vi "niScope Get Capabilities.vi"(8 "error in":errorcluster, 10 "fs [Hz]":dbl, 11 "niScope session in":T2={"channel cfg"=[], "sessions"=[], "multi cards"=FALSE, "channels"=0, "type"=enum."n/a", "memory [B/chn]"=0, "ext. clock [Hz]"=0.0, "samples count"=0, "use streaming"=FALSE, "proc setup"={"packet size [smpl]"=0, "current timeout [s]"=0.0, "blk2blk timeout [s]"=0.0, "event time"=timestamp(0 s since 1904-01-01), "temp sampl T [s]"=0.0, "data queue"=refnum, "stop notifier"=refnum, "proc ref"=refnum}, "sample width [B]"=0, "ranges [V]"=[], "trigger setup"={"coupling"=1, "level [V]"=0.0, "slope"=0, "mode"=enum."Immediate"}, "fs [Hz]"=0.0} {"trigger setup"."level [V]" format="%.2f"; "trigger setup"."coupling" items=["AC"=0, "DC"=1, "HF Reject"=3, "LF Reject"=4, "AC Plus HF Reject"=1001]; "channel cfg"."Range [Vpk]" min=0.0; "channel cfg"."Channel" min=0}) -> (0 "error out":errorcluster, 2 "capabilities":T1, 3 "niScope session out":T2={"channel cfg"=[], "sessions"=[], "multi cards"=FALSE, "channels"=0, "type"=enum."n/a", "memory [B/chn]"=0, "ext. clock [Hz]"=0.0, "samples count"=0, "use streaming"=FALSE, "proc setup"={"packet size [smpl]"=0, "current timeout [s]"=0.0, "blk2blk timeout [s]"=0.0, "event time"=timestamp(0 s since 1904-01-01), "temp sampl T [s]"=0.0, "data queue"=refnum, "stop notifier"=refnum, "proc ref"=refnum}, "sample width [B]"=0, "ranges [V]"=[], "trigger setup"={"coupling"=1, "level [V]"=0.0, "slope"=0, "mode"=enum."Immediate"}, "fs [Hz]"=0.0} {"trigger setup"."level [V]" format="%.2f"; "trigger setup"."coupling" items=["AC"=0, "DC"=1, "HF Reject"=3, "LF Reject"=4, "AC Plus HF Reject"=1001]; "channel cfg"."Range [Vpk]" min=0.0; "channel cfg"."Channel" min=0})   [LabVIEW 2013, in "niScope Virtual Digitizer.lvlib"]
doc: "This will return capabilities of selected HW. To make it work the session must contain valid setup of the channels and must also contain output of the 'Initialize Virtual Channels' VI, i.e. it may be calle either within opened session or even after the session was closed, because the data produced by 'Initialize Virtual Channels' stay in the session."
uses:
  niScope Virtual Digitizer.lvlib
  niScope Session.ctl
  niScope Virtual Channel Config.ctl
  niScope Virtual Channel Mode.ctl
  niScope Virtual Channel Input Z.ctl
  niScope Virtual Channel Coupling.ctl
  niScope Type.ctl
  niScope Digitizing Process Options.ctl
  niScope Data Packet.ctl
  niScope Trigger Setup.ctl
  <instrlib>/niScope/Controls/niScope trigger coupling.ctl
  <instrlib>/niScope/Controls/niScope trigger slope.ctl
  niScope Capabilities.ctl
  <vilib>/Utility/error.llb/Error Cluster From Error Code.vi
  <vilib>/ErrorRing/Error Ring.xnode
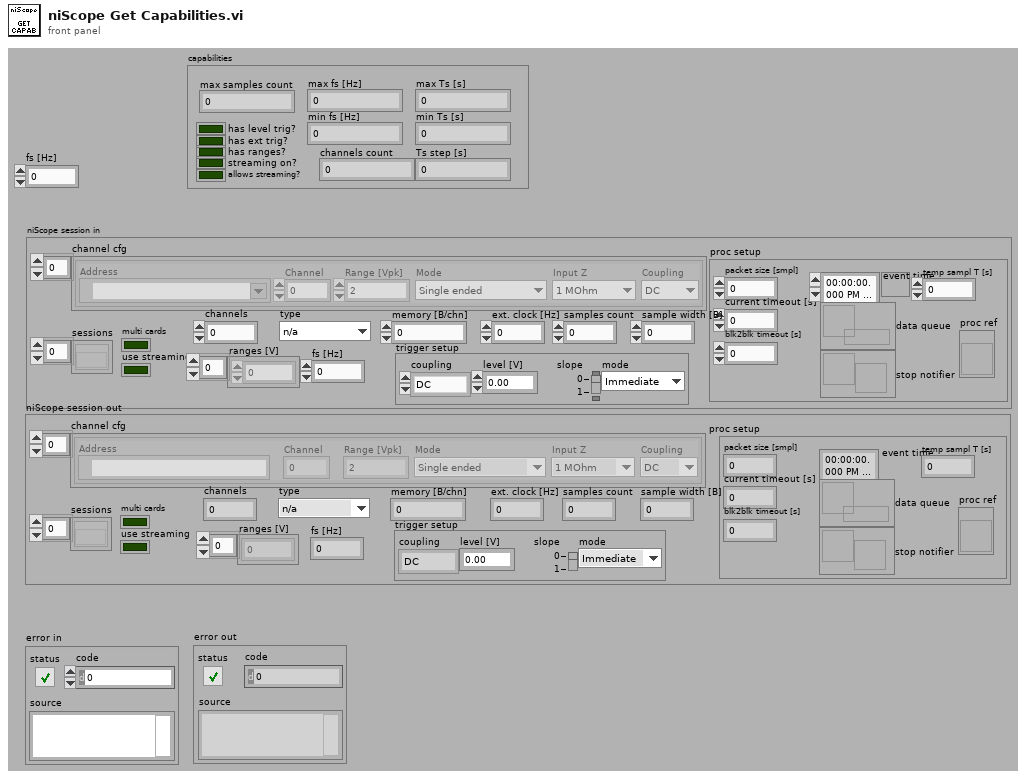
[diagram p1: front panel]
types:
  T1 = typedef "niScope Virtual Digitizer.lvlib/niScope Capabilities.ctl" = cluster{"max samples count":i64, "max fs [Hz]":ext, "min fs [Hz]":ext, "Ts step [s]":ext, "max Ts [s]":ext, "min Ts [s]":ext, "allows streaming?":bool, "streaming on?":bool, "has level trig?":bool, "has ext trig?":bool, "channels count":i32, "has ranges?":bool}
  T2 = typedef "niScope Virtual Digitizer.lvlib/niScope Session.ctl" = cluster{"channel cfg":T3[], "sessions":refnum<k20>[], "multi cards":bool, "channels":i32, "type":T7, "memory [B/chn]":i32, "ext. clock [Hz]":dbl, "samples count":i64, "use streaming":bool, "proc setup":T8, "sample width [B]":i32, "ranges [V]":dbl[], "trigger setup":T9, "fs [Hz]":dbl}
  T3 = typedef "niScope Virtual Digitizer.lvlib/niScope Virtual Channel Config.ctl" = cluster{"Address":refnum<k15>, "Channel":i32, "Mode":T4, "Input Z":T5, "Coupling":T6, "Range [Vpk]":dbl}
  T4 = typedef "niScope Virtual Digitizer.lvlib/niScope Virtual Channel Mode.ctl" = enum16{"Single ended", "Unbal. differential", "Differential"}
  T5 = typedef "niScope Virtual Digitizer.lvlib/niScope Virtual Channel Input Z.ctl" = enum16{"1 MOhm", "50 Ohm"}
  T6 = typedef "niScope Virtual Digitizer.lvlib/niScope Virtual Channel Coupling.ctl" = enum16{"AC", "DC", "GND"}
  T7 = typedef "niScope Virtual Digitizer.lvlib/niScope Type.ctl" = enum16{"n/a", "5922"}
  T8 = typedef "niScope Virtual Digitizer.lvlib/niScope Digitizing Process Options.ctl" = cluster{"packet size [smpl]":i64, "current timeout [s]":dbl, "blk2blk timeout [s]":dbl, "event time":timestamp, "temp sampl T [s]":dbl, "data queue":refnum<queue>, "stop notifier":refnum<notifier>, "proc ref":refnum<vi>}
  T9 = typedef "niScope Virtual Digitizer.lvlib/niScope Trigger Setup.ctl" = cluster{"coupling":T10, "level [V]":dbl, "slope":T11, "mode":enum16{"Immediate", "External", "Level"}}
  T10 = typedef "niScope trigger coupling.ctl" = u16
  T11 = typedef "niScope trigger slope.ctl" = i32
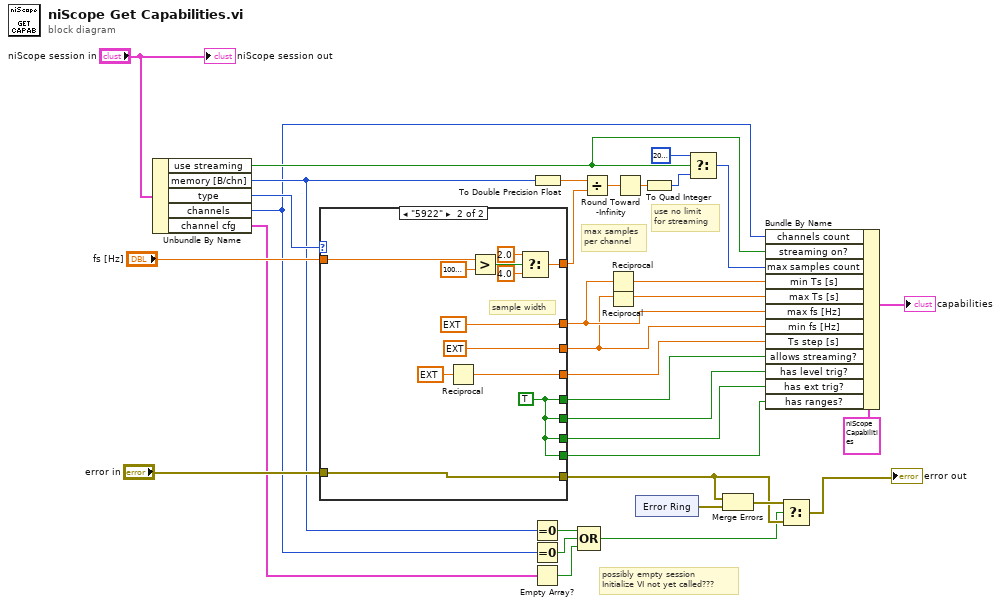
[diagram p0: block diagram]
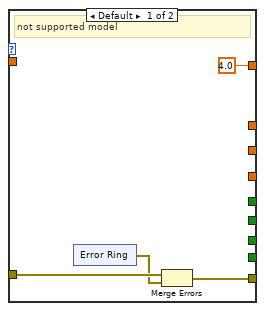
[diagram p2: hidden frame]
diagram:
  # "possibly empty session\nInitialize VI not yet called???"
  # "use no limit\nfor streaming"
  # "max samples\nper channel"
  n1 = Unbundle By Name("niScope session in") -> ("use streaming"=w18:bool, "memory [B/chn]"=w10:i32, "type"=w33:T7, "channels"=w2:i32, "channel cfg"=w9:T3[])
  n2 = case shown="\"5922\"" w33 {
    tunnel: "fs [Hz]" -> [_ w55]
    tunnel: [4.0 ("t") w50] -> w31
    tunnel: [_ ext 15000000.0 ("y")] -> w22
    tunnel: [_ ext 50000.0 ("y")] -> w21
    tunnel: [_ w46] -> w20
    tunnel: [_ w44] -> w19
    tunnel: "error in" -> [w37 w45]
    tunnel: [w36 w45] -> w12
    tunnel: [_ w44] -> w4
    tunnel: [_ w44] -> w3
    tunnel: [_ w44] -> w1
    frame Default {
      # "not supported model"
      n3 = xnode "Error Ring"() -> ("error out"=w35:errorcluster)
      n4 = Merge Errors(w37, w35) -> (w36:errorcluster)
    }
    frame "5922" {
      w44 = TRUE
      # "sample width"
      n5 = Reciprocal(x=ext 60000000.0 ("y")) -> (1/x=w46:ext)
      n6 = Greater?(x=w55, y=10000000.0) -> (0:w53:bool)
      n7 = Select(t=2.0, s=w53, f=4.0 ("t")) -> (s? t:f=w50:dbl)
    }
  }
  n8 = Equal To 0?(x=w10) -> (x = 0?=w8:bool)
  n9 = Equal To 0?(x=w2) -> (x = 0?=w7:bool)
  n10 = Empty Array?(array=w9) -> (empty?=w6:bool)
  n11 = To Double Precision Float(number=w10) -> (double precision float=w32:dbl)
  n12 = Compound Arithmetic op=OR(w8, w7, w6) -> (w5:bool)
  n13 = Divide(x=w32, y=w31) -> (x/y=w30:dbl)
  n14 = Reciprocal(x=w22) -> (1/x=w24:ext)
  n15 = Reciprocal(x=w21) -> (1/x=w23:ext)
  n16 = Round Toward -Infinity(1:w30) -> (0:w29:dbl)
  n17 = xnode "Error Ring"() -> ("error out"=w11:errorcluster)
  n18 = To Quad Integer(1:w29) -> (0:w28:i64)
  n19 = Select(t=i64 2000000000, s=w18, f=w28) -> (s? t:f=w25:i64)
  n20 = Merge Errors(w12, w11) -> (w13:errorcluster)
  n21 = Bundle By Name(cluster=T1 {"max samples count"=0, "max fs [Hz]"=0.0, "min fs [Hz]"=0.0, "Ts step [s]"=0.0, "max Ts [s]"=0.0, "min Ts [s]"=0.0, "allows streaming?"=FALSE, "streaming on?"=FALSE, "has level trig?"=FALSE, "has ext trig?"=FALSE, "channels count"=0, "has ranges?"=FALSE} ("capabilities"), "channels count"=w2, "streaming on?"=w18, "max samples count"=w25, "min Ts [s]"=w24, "max Ts [s]"=w23, "max fs [Hz]"=w22, "min fs [Hz]"=w21, "Ts step [s]"=w20, "allows streaming?"=w19, "has level trig?"=w4, "has ext trig?"=w3, "has ranges?"=w1) -> (→"capabilities":T1)
  n22 = Select(t=w13, s=w5, f=w12) -> (s? t:f=→"error out":errorcluster)
  "niScope session out" <- "niScope session in"
